vi "wyswietlInfoOZrealizowanychPunktach.vi"(5 "Lista punktow":i32[](array[numeric])) -> ()   [LabVIEW 2014]
uses:
  AkcjaGFV.ctl
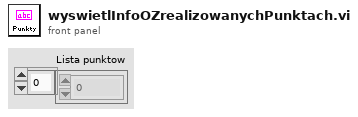
[diagram p1: front panel]
types:
  T1 = typedef "AkcjaGFV.ctl" = enum16{"Czytaj", "Zapisz", "Reset"}
  T2 = typedef "WyjsciaParametry.ctl" = cluster{"Nad. lewo":bool, "Nad.  prawo":bool, "Nad.  góra":bool, "Nad. dół":bool, "Działanie":bool, "Pomiar":bool, "Odb. dół":bool, "Odb.  góra":bool, "Odb.  prawo":bool, "Odb. lewo":bool, "Punkty pom. info":string}
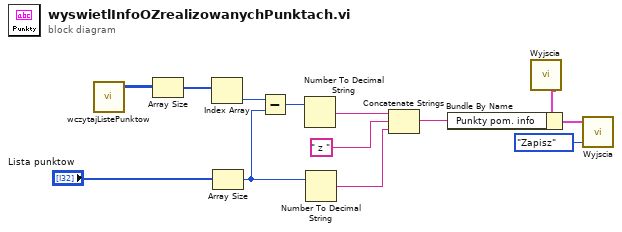
[diagram p0: block diagram]
diagram:
  n1 = call "wczytajListePunktow.vi"() -> ("Wspolrzedne katowe"=w13:i32[][])  [unwired: 5 in]
  n2 = Array Size(array=w13) -> (size(s)=w12:i32[])
  n3 = Index Array(array=w12) -> (element=w11:i32)  [unwired: 1 in]
  n4 = Array Size(array="Lista punktow") -> (size(s)=w9:i32)
  n5 = Subtract(x=w11, y=w9) -> (x-y=w10:i32)
  n6 = Number To Decimal String(number=w10) -> (decimal integer string=w8:string)  [unwired: 1 in]
  n7 = Number To Decimal String(number=w9) -> (decimal integer string=w7:string)  [unwired: 1 in]
  n8 = Concatenate Strings(w8, " z " ("string"), w7) -> (w4:string)
  n9 = call "Wyjscia.vi"() -> ("Wyjście"=w5:T2)  [unwired: 5 in]
  n10 = Bundle By Name(cluster=w5, "Punkty pom. info"=w4) -> (w3:T2)
  n11 = call "Wyjscia.vi"("Akcja"=AkcjaGFV."Zapisz", "Wejście"=w3) -> ()  [unwired: 3 in, 1 out]
